vi "DW_add.vi"(3 "dizhi":string, 5 "quxian":string, 6 "city":string, 7 "LabVIEW Web Service Request":refnum<class "Web Request.lvclass"> caption="LabVIEW Web服务请求", 8 "sheng":string, 9 "id":string, 10 "name":string, 11 "action":string) -> (0 "error out 2":errorcluster, 1 "data2":string[][](array[string]) caption="查询数据")   [LabVIEW 2017]
uses:
  <vilib>/wsapi/Web Request.lvclass
panel:
  out "postdata":string caption="post数据"
  out "error out":errorcluster caption="错误输出"
  # "Web服务请求输入接线端用于调用“Web服务”选板的VI。除非不需要访问该选板，否则不要在连线板上删除这个输入接线端。"
  # "添加至连线板的每一个其他输入控件，在URL中对应于一个输入。如需在接线端模式输出（默认设置）下包含显示控件，则该显示控件必须与连线板相连。"
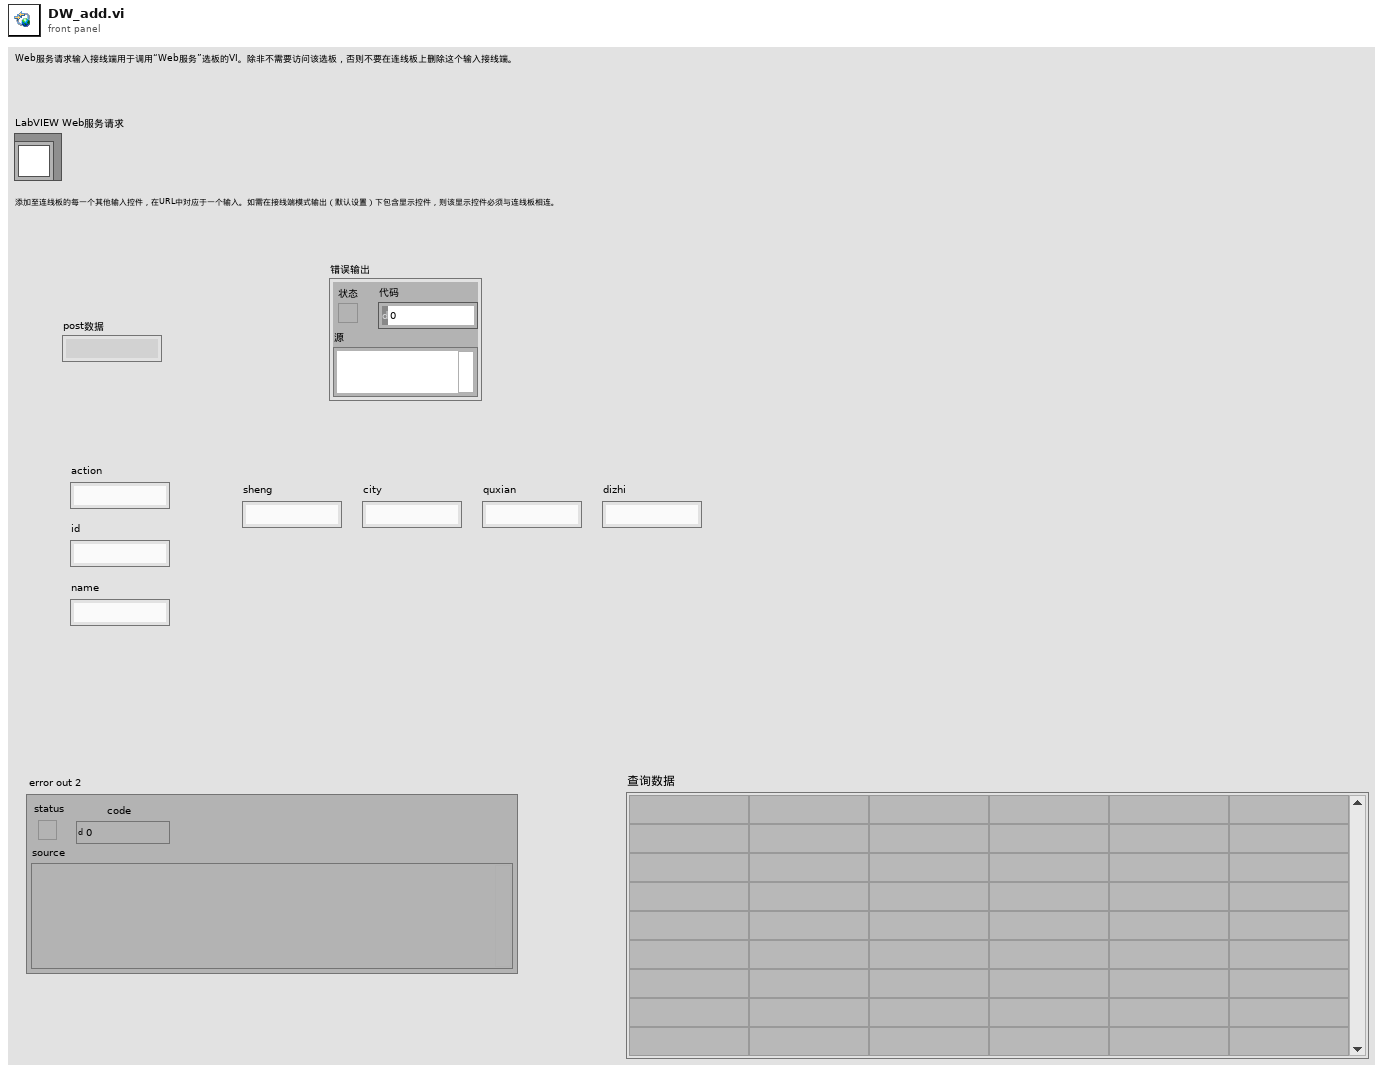
[diagram p1: front panel]
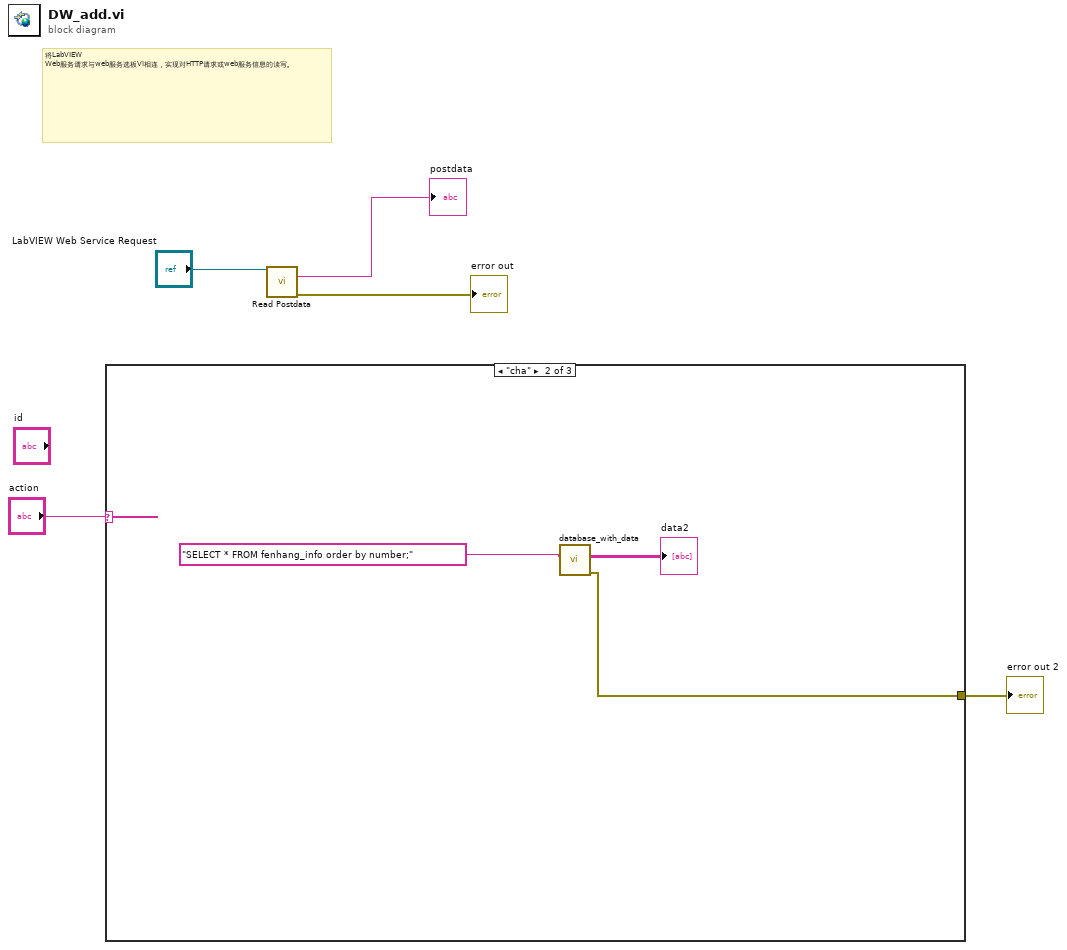
[diagram p0: block diagram]
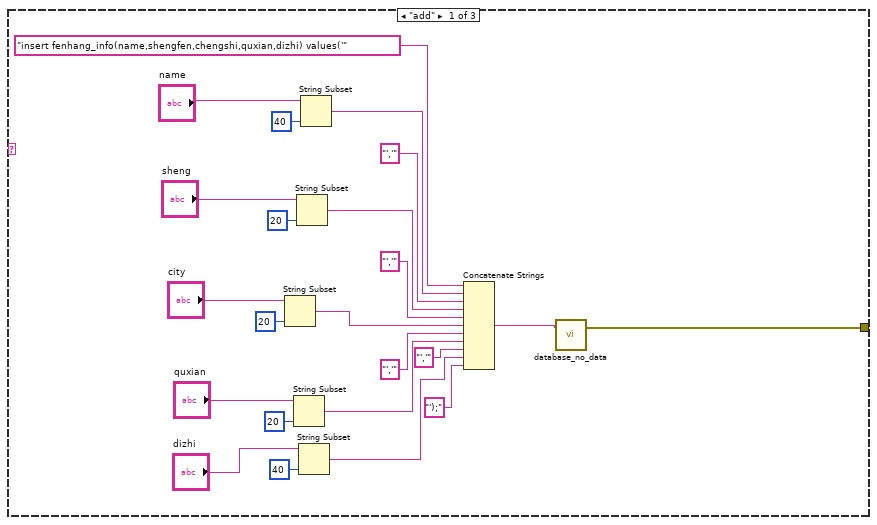
[diagram p2: hidden frame]
diagram:
  # "将LabVIEW Web服务请求与web服务选板VI相连，实现对HTTP请求或web服务信息的读写。"
  n1 = case shown="\"cha\"" "action" {
    tunnel: [w6 w29 _] -> w1
    frame "add" {
      n2 = String Subset(string="city", length (rest)=20 ("长度（剩余）")) -> (substring=w20:string)  [unwired: 1 in]
      n3 = String Subset(string="quxian", length (rest)=20 ("长度（剩余）")) -> (substring=w18:string)  [unwired: 1 in]
      n4 = String Subset(string="sheng", length (rest)=20 ("长度（剩余）")) -> (substring=w22:string)  [unwired: 1 in]
      n5 = String Subset(string="dizhi", length (rest)=40 ("长度（剩余）")) -> (substring=w9:string)  [unwired: 1 in]
      n6 = String Subset(string="name", length (rest)=40 ("长度（剩余）")) -> (substring=w24:string)  [unwired: 1 in]
      n7 = Concatenate Strings("insert fenhang_info(name,shengfen,chengshi,quxian,dizhi) values('" ("格式字符串"), w24, "','" ("字符串"), w22, "','" ("字符串"), w20, "','" ("字符串"), w18, "','" ("字符串"), w9, "');" ("字符串")) -> (w7:string)
      n8 = call "database_no_data.vi"("input"=w7) -> ("error"=w6:errorcluster)  [unwired: 2 in]
    }
    frame "cha" {
      n9 = call "database_with_data.vi"("input"="SELECT * FROM fenhang_info order by number;" ("格式字符串")) -> ("error"=w29:errorcluster, "Data"=→"data2":string[][])  [unwired: 9 in]
    }
    frame Default {
    }
  }
  "error out 2" <- w1
  n10 = call <vilib>:"Read Postdata.vi"("LabVIEW Web Service Request"="LabVIEW Web Service Request") -> ("postdata"=→"postdata":string, "error out"=→"error out":errorcluster)  [unwired: 12 in, 1 out]
